vi "Get Display Image.vi"(8 "error in (no error)":errorcluster, 11 "SerializableObject in":refnum<class "SerializableObject.lvclass">) -> (0 "error out":errorcluster, 2 "Image":picture, 3 "SerializableObject out":refnum<class "SerializableObject.lvclass">)   [LabVIEW 2015, in "SerializableObject.lvclass"]
uses:
  SerializableObject.lvclass
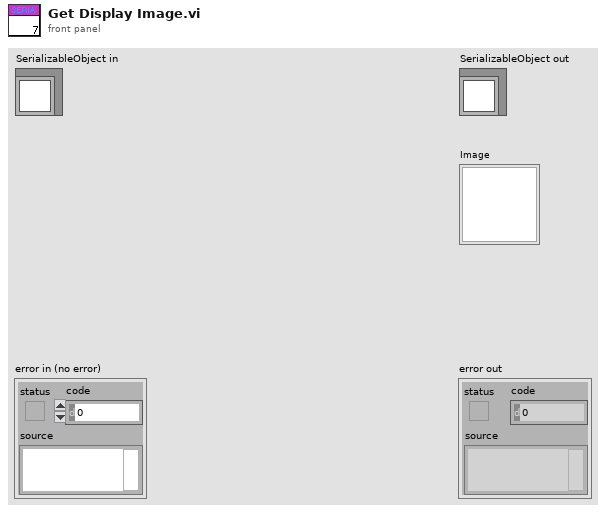
[diagram p1: front panel]
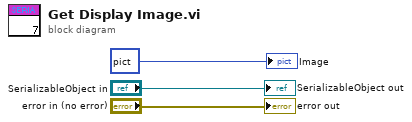
[diagram p0: block diagram]
diagram:
  "error out" <- "error in (no error)"
  "SerializableObject out" <- "SerializableObject in"
  "Image" <- picture bytes[782] ("Image")
